vi "testset.vi"() -> ()   [LabVIEW 2019, in "SpectraPro.lvlib"]
uses:
  SpectraPro.lvlib
panel:
  out "read buffer 13":string
  out "read buffer 12":string
  out "read buffer 11":string
  out "read buffer 10":string
  out "read buffer 9":string
  out "read buffer 8":string
  out "read buffer 7":string
  out "read buffer 6":string
  out "read buffer 5":string
  out "read buffer 4":string
  out "read buffer 2":string
  out "read buffer":string
  out "set grating id":i32
  out "initial grating id":i32
  out "set wavelength":dbl
  out "initial wavelength":dbl
  out "set slit width":i32
  out "initial slit width":i32
  in  "VISA resource name":refnum<visa-resource-name>="COM9"
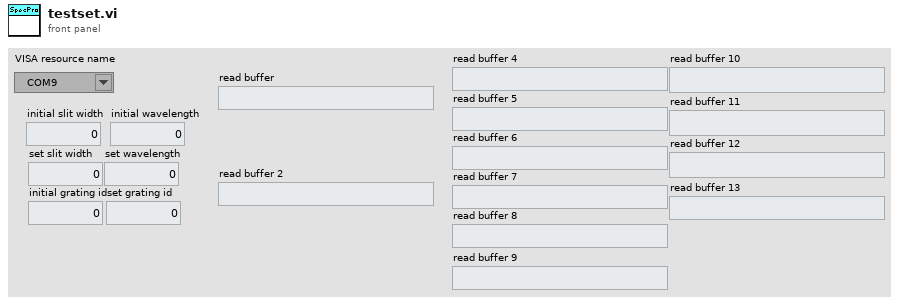
[diagram p1: front panel]
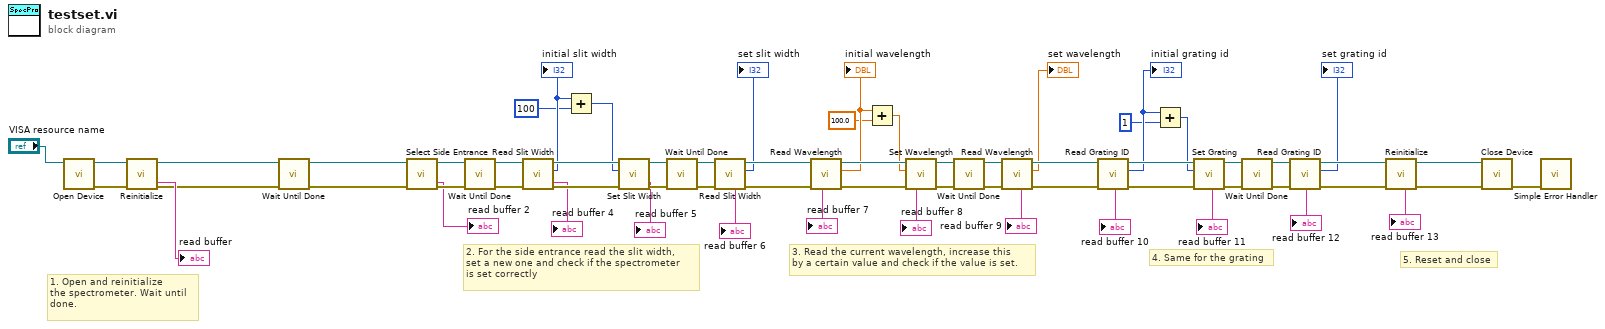
[diagram p0: block diagram]
diagram:
  # "5. Reset and close"
  # "4. Same for the grating"
  # "3. Read the current wavelength, increase this\nby a certain value and check if the value is set."
  # "2. For the side entrance read the slit width,\nset a new one and check if the spectrometer\nis set correctly"
  # "1. Open and reinitialize\nthe spectrometer. Wait until\ndone."
  n1 = call "Open Device.vi"("VISA resource name"="VISA resource name") -> ("error out"=w60:errorcluster, "VISA resource name out"=w62:refnum<visa-resource-name>)  [unwired: 9 in]
  n2 = call "Reinitialize.vi"("error in (no error)"=w60, "VISA resource name"=w62) -> ("error out"=w4:errorcluster, "VISA resource name out"=w2:refnum<visa-resource-name>, "read buffer"=→"read buffer":string)  [unwired: 7 in]
  n3 = call "Wait Until Done.vi"("error in (no error)"=w4, "VISA resource name"=w2) -> ("error out"=w3:errorcluster, "VISA resource name out"=w1:refnum<visa-resource-name>)  [unwired: 8 in]
  n4 = call "Select Side Entrance.vi"("error in (no error)"=w3, "VISA resource name"=w1) -> ("error out"=w59:errorcluster, "VISA resource name out"=w15:refnum<visa-resource-name>, "read buffer"=→"read buffer 2":string)  [unwired: 7 in]
  n5 = call "Wait Until Done.vi"("error in (no error)"=w59, "VISA resource name"=w15) -> ("error out"=w16:errorcluster, "VISA resource name out"=w14:refnum<visa-resource-name>)  [unwired: 8 in]
  n6 = call "Read Slit Width.vi"("error in (no error)"=w16, "VISA resource name"=w14) -> ("error out"=w58:errorcluster, "Slit Width (um)"=w41:i32, "VISA resource name out"=w48:refnum<visa-resource-name>, "read buffer"=→"read buffer 4":string)  [unwired: 6 in]
  "initial slit width" <- w41
  n7 = Add(x=w41, y=100) -> (x+y=w39:i32)
  n8 = call "Set Slit Width.vi"("error in (no error)"=w58, "Slit Width (um)"=w39, "VISA resource name"=w48) -> ("error out"=w57:errorcluster, "VISA resource name out"=w12:refnum<visa-resource-name>, "read buffer"=→"read buffer 5":string)  [unwired: 6 in]
  n9 = call "Wait Until Done.vi"("error in (no error)"=w57, "VISA resource name"=w12) -> ("error out"=w13:errorcluster, "VISA resource name out"=w11:refnum<visa-resource-name>)  [unwired: 8 in]
  n10 = call "Read Slit Width.vi"("error in (no error)"=w13, "VISA resource name"=w11) -> ("error out"=w56:errorcluster, "Slit Width (um)"=→"set slit width":i32, "VISA resource name out"=w47:refnum<visa-resource-name>, "read buffer"=→"read buffer 6":string)  [unwired: 6 in]
  n11 = call "Read Wavelength.vi"("error in (no error)"=w56, "VISA resource name"=w47) -> ("error out"=w55:errorcluster, "Wavelength (nm)"=w36:dbl, "VISA resource name out"=w46:refnum<visa-resource-name>, "read buffer"=→"read buffer 7":string)  [unwired: 6 in]
  "initial wavelength" <- w36
  n12 = Add(x=w36, y=100.0) -> (x+y=w34:dbl)
  n13 = call "Set Wavelength.vi"("error in (no error)"=w55, "Wavelength (nm)"=w34, "VISA resource name"=w46) -> ("error out"=w54:errorcluster, "VISA resource name out"=w9:refnum<visa-resource-name>, "read buffer"=→"read buffer 8":string)  [unwired: 6 in]
  n14 = call "Wait Until Done.vi"("error in (no error)"=w54, "VISA resource name"=w9) -> ("error out"=w10:errorcluster, "VISA resource name out"=w8:refnum<visa-resource-name>)  [unwired: 8 in]
  n15 = call "Read Wavelength.vi"("error in (no error)"=w10, "VISA resource name"=w8) -> ("error out"=w53:errorcluster, "Wavelength (nm)"=→"set wavelength":dbl, "VISA resource name out"=w45:refnum<visa-resource-name>, "read buffer"=→"read buffer 9":string)  [unwired: 6 in]
  n16 = call "Read Grating ID.vi"("error in (no error)"=w53, "VISA resource name"=w45) -> ("error out"=w52:errorcluster, "Grating ID"=w31:i32, "VISA resource name out"=w44:refnum<visa-resource-name>, "read buffer"=→"read buffer 10":string)  [unwired: 6 in]
  "initial grating id" <- w31
  n17 = Add(x=w31, y=1) -> (x+y=w32:i32)
  n18 = call "Set Grating.vi"("error in (no error)"=w52, "Grating ID"=w32, "VISA resource name"=w44) -> ("error out"=w51:errorcluster, "VISA resource name out"=w6:refnum<visa-resource-name>, "read buffer"=→"read buffer 11":string)  [unwired: 6 in]
  n19 = call "Wait Until Done.vi"("error in (no error)"=w51, "VISA resource name"=w6) -> ("error out"=w7:errorcluster, "VISA resource name out"=w5:refnum<visa-resource-name>)  [unwired: 8 in]
  n20 = call "Read Grating ID.vi"("error in (no error)"=w7, "VISA resource name"=w5) -> ("error out"=w50:errorcluster, "Grating ID"=→"set grating id":i32, "VISA resource name out"=w43:refnum<visa-resource-name>, "read buffer"=→"read buffer 12":string)  [unwired: 6 in]
  n21 = call "Reinitialize.vi"("error in (no error)"=w50, "VISA resource name"=w43) -> ("error out"=w49:errorcluster, "VISA resource name out"=w42:refnum<visa-resource-name>, "read buffer"=→"read buffer 13":string)  [unwired: 7 in]
  n22 = call "Close Device.vi"("error in (no error)"=w49, "VISA resource name"=w42) -> ("error out"=w27:errorcluster)  [unwired: 9 in]
  n23 = call <vilib>:"Simple Error Handler.vi"("error in (no error)"=w27) -> ()  [unwired: 4 in, 5 out]
